vi "Initialize Addon.vi"(8 "error in (no error)":errorcluster, 11 "Cluster":T19={"J1939 XNET Settings"={"XNET Database"="", "XNET Cluster"="", "CAN Port"="", "Baud rate [Bd]"=0, "Termination"=0, "Incoming Rate"=0, "Outcoming Rate"=0, "Write Decimation"=1}, "Incoming Decimation"=0, "Outgoing Decimation"=0, {"RT Bitfile Path"=path "", "RIO Device"=0, "Enable"=FALSE}, "Incoming Single Point Configuraiton"={"Incoming Single Point Frame"={"ID"=[], "Channel Array Positions"=[], "Frame Length"=[], "Frame Channels"=[]}, "Channel Pairs"={"Chan Refs"=[], "Previous Chan Values"=[]}, "# of Channels"=0, "Name"=""}, "Outgoing Cyclic Configuraiton"={"Outgoing Cyclic Frame"={"ID"=[], "Channel Array Positions"=[], "Frame Length"=[], "Transmit Propreties"=[], "Frame Channels"=[]}, "Channel Pairs"={"Block Data Refs"=[], "Previous Chan Values"=[]}, "Name"=""}, "Internal Command Engine References"={"Response Refs"={"Block Data Refs"=[], "Values Array"=[], "# of Channels"=0, "Name"=""}, "Command Refs"={"Block Data Refs"=[], "Values Array"=[], "# of Channels"=0, "Name"=""}, "Command Names"=[], "Response Names"=[]}, "FPGA Bitfile Settings"={"RT Bitfile Path"=path "", "RIO Device"=0, "Enable"=FALSE}, "J1939 Monitor Settings"={"J1939 Network Address"=0, "Name"=0}, "Simulated Addresses"=[]} {"Simulated Addresses"."J1939 XNET Settings"."Name" format="%.0x"; "Simulated Addresses"."DM1 Data"."Data Reference" format="%.0x"; "Simulated Addresses"."DM1 Active?"."Data Reference" format="%.0x"; "Simulated Addresses"."DM2 Data"."Data Reference" format="%.0x"; "Simulated Addresses"."DM2 Active?"."Data Reference" format="%.0x"; "J1939 Monitor Settings"."Name" format="%.0x"; "J1939 XNET Settings"."Termination" items=["Off", "On"]; "Incoming Single Point Configuraiton"."Channel Pairs"."Chan Refs" format="%.0x"; "Outgoing Cyclic Configuraiton"."Outgoing Cyclic Frame"."Transmit Propreties"."Transmit Time" format="%#_p"; "Outgoing Cyclic Configuraiton"."Channel Pairs"."Block Data Refs"."Data Reference" format="%.0x"; "Internal Command Engine References"."Response Refs"."Block Data Refs" format="%.0x"; "Internal Command Engine References"."Command Refs"."Block Data Refs"."Data Reference" format="%.0x"}) -> (0 "error out":errorcluster, 3 "cluster":T1={"Device Error"={"status"=FALSE, "code"=0, "source"=""}, "VI Refs"=[], "Error Handling Cluster"={"Error Process Q"=refnum, "Process Qs"=[]}, "J1939 Process Parameters"={"J1939 XNET Settings"={"XNET Database"="", "XNET Cluster"="", "CAN Port"="", "Baud rate [Bd]"=0, "Termination"=0, "Incoming Rate"=0, "Outcoming Rate"=1, "Write Decimation"=1}, "Incoming Single Point Configuraiton"={"Incoming Single Point Frame"={"ID"=[], "Conversion"=[], "Channel Array Positions"=[], "Frame Length"=[]}, "Channel Pairs"={"Chan Refs"=[], "Previous Chan Values"=[]}, "Read FIFO"=refnum}, "Outgoing Cyclic Configuraiton"={"Outgoing Cyclic Frame"={"ID"=[], "Conversion"=[], "Channel Array Positions"=[], "Frame Length"=[], "Transmit Propreties"=[]}, "Channel Pairs"={"Block Data Refs"=[], "Previous Chan Values"=[]}, "Write FIFO"=refnum}, "J1939 Monitor Settings"={"J1939 Network Address"=0, "Name"=0}, "Simulated Addresses"=[], "Simulated Addresses LUT"=variant}, "Internal Command Engine References"={"Response Refs"={"Block Data Refs"=[], "Values Array"=[]}, "Command Refs"={"Block Data Refs"=[], "Values Array"=[]}, "Response HW_Internal Cmds"=refnum, "Command HW_Internal Cmds"=refnum, "Command Names"=[], "Response Names"=[]}, "FPGA Session"=0, "Incoming Decimation"=0, "Outgoing Decimation"=0} {"Internal Command Engine References"."Command Refs"."Block Data Refs"."Data Reference" format="%.0x"; "Internal Command Engine References"."Response Refs"."Block Data Refs" format="%.0x"; "J1939 Process Parameters"."Simulated Addresses"."Simulated Addresses"."J1939 XNET Settings"."Name" format="%.0x"; "J1939 Process Parameters"."J1939 Monitor Settings"."Name" format="%.0x"; "J1939 Process Parameters"."Outgoing Cyclic Configuraiton"."Channel Pairs"."Block Data Refs"."Data Reference" format="%.0x"; "J1939 Process Parameters"."Outgoing Cyclic Configuraiton"."Outgoing Cyclic Frame"."Transmit Propreties"."Transmit Time" format="%#_p"; "J1939 Process Parameters"."J1939 XNET Settings"."Termination" items=["Off", "On"]; "J1939 Process Parameters"."Incoming Single Point Configuraiton"."Channel Pairs"."Chan Refs" format="%.0x"})   [LabVIEW 2013, in "J1939 Addon Engine.lvlib"]
uses:
  J1939 Addon Engine.lvlib
  Shared/Types/Compile Addon Settings.ctl
  Shared/Types/XNET Settings.ctl
  Shared/Types/SysDef FPGA Settings.ctl
  Shared/Types/SysDef Incoming Single Point Configurations.ctl
  Shared/Types/SysDef Incoming Frame Configuration.ctl
  Types/Incoming Single Point Channel Pairs.ctl
  <vilib>/NI Veristand/Custom Device API/Data Reference.ctl
  Shared/Types/SysDef Outgoing Cyclic Configurations.ctl
  Shared/Types/SysDef Outgoing Frame Configuration.ctl
  Shared/Types/XNET Frame Event Properties.ctl
  Types/Outgoing Cyclic Channel Pairs.ctl
  <vilib>/NI Veristand/Custom Device API/Block Data Reference.ctl
  Shared/Types/SysDef Command Settings.ctl
  Shared/Types/Monitor Settings.ctl
  Shared/Types/Compiled Simulated Settings.ctl
  Types/Inline Device Cluster.ctl
  Error Handling API/Controls/Error Handling Cluster.ctl
  Types/Process Parameters.ctl
  Types/Incoming Single Point Configuration.ctl
  Types/Incoming Single Point Frame Pairs.ctl
  Types/Outgoing Cyclic Configuration.ctl
  Types/Outgoing Cyclic Frame Pairs.ctl
  Types/Simulated Settings.ctl
  Types/DTC FIFOs.ctl
  Types/Internal Command Configuration Parameters.ctl
  <vilib>/NI Veristand/Custom Device API/Custom Device API.lvlib
  Shared/J1939 Addon Shared.lvlib
  Error Handling API/Error Handling API.lvlib
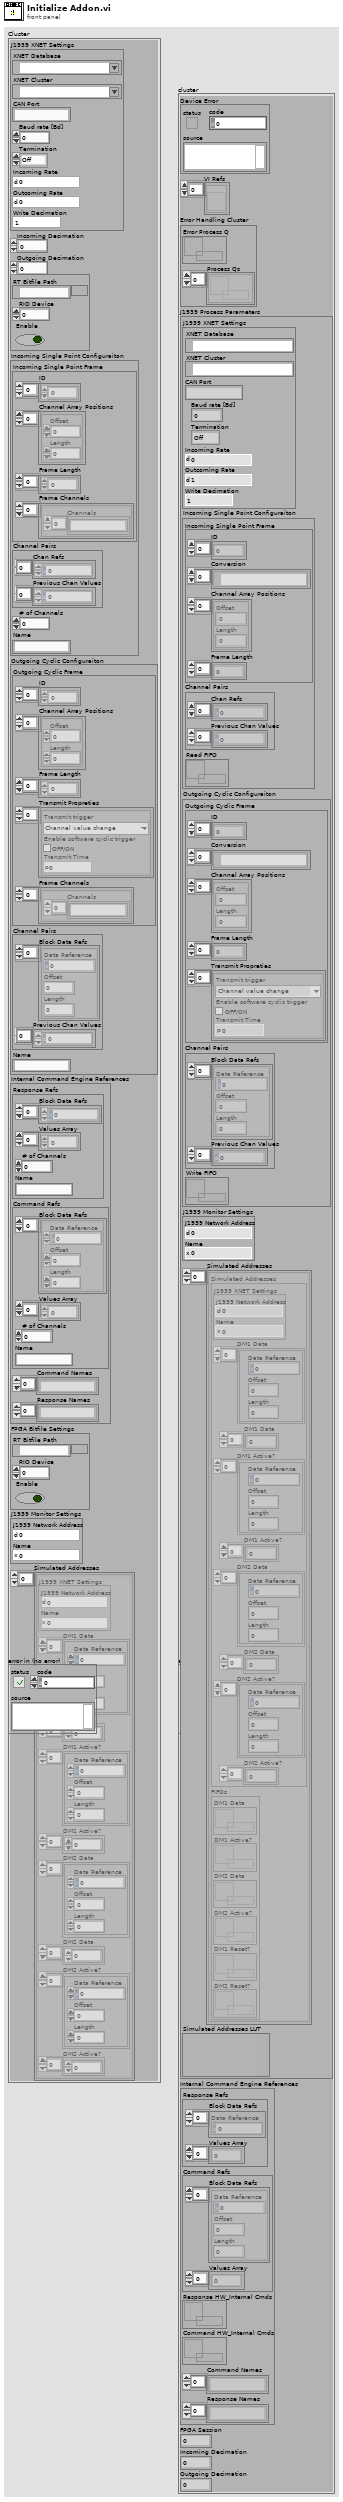
[diagram p1: front panel]
types:
  T1 = typedef "J1939 Addon Engine.lvlib/Inline Device Cluster.ctl" = cluster{"Device Error":errorcluster, "VI Refs":refnum<vi>[], "Error Handling Cluster":T2, "J1939 Process Parameters":T3, "Internal Command Engine References":T18, "FPGA Session":u32, "Incoming Decimation":u32, "Outgoing Decimation":u32}
  T2 = typedef "J1939 Addon Engine.lvlib/Error Handling API.lvlib/Error Handling Cluster.ctl" = cluster{"Error Process Q":refnum<queue>, "Process Qs":refnum<queue>[]}
  T3 = typedef "J1939 Addon Engine.lvlib/Process Parameters.ctl" = cluster{"J1939 XNET Settings":T4, "Incoming Single Point Configuraiton":T5, "Outgoing Cyclic Configuraiton":T9, "J1939 Monitor Settings":T14, "Simulated Addresses":T15[], "Simulated Addresses LUT":variant}
  T4 = typedef "J1939 Addon Shared.lvlib/XNET Settings.ctl" = cluster{"XNET Database":refnum<k21>, "XNET Cluster":refnum<k21>, "CAN Port":string, "Baud rate [Bd]":u32, "Termination":u32, "Incoming Rate":u32, "Outcoming Rate":u32, "Write Decimation":u32}
  T5 = typedef "J1939 Addon Engine.lvlib/Incoming Single Point Configuration.ctl" = cluster{"Incoming Single Point Frame":T6, "Channel Pairs":T7, "Read FIFO":refnum<k33>}
  T6 = typedef "J1939 Addon Engine.lvlib/Incoming Single Point Frame Pairs.ctl" = cluster{"ID":u32[], "Conversion":refnum<k21>[], "Channel Array Positions":cluster{"Offset":u32, "Length":u32}[], "Frame Length":u32[]}
  T7 = typedef "J1939 Addon Engine.lvlib/Incoming Single Point Channel Pairs.ctl" = cluster{"Chan Refs":T8[], "Previous Chan Values":dbl[]}
  T8 = typedef "Custom Device API.lvlib/Data Reference.ctl" = i32
  T9 = typedef "J1939 Addon Engine.lvlib/Outgoing Cyclic Configuration.ctl" = cluster{"Outgoing Cyclic Frame":T10, "Channel Pairs":T12, "Write FIFO":refnum<k33>}
  T10 = typedef "J1939 Addon Engine.lvlib/Outgoing Cyclic Frame Pairs.ctl" = cluster{"ID":u32[], "Conversion":refnum<k21>[], "Channel Array Positions":cluster{"Offset":u32, "Length":u32}[], "Frame Length":u32[], "Transmit Propreties":T11[]}
  T11 = typedef "J1939 Addon Shared.lvlib/XNET Frame Event Properties.ctl" = cluster{"Transmit trigger":enum16{"Channel value change"}, "Enable software cyclic trigger":bool, "Transmit Time":dbl}
  T12 = typedef "J1939 Addon Engine.lvlib/Outgoing Cyclic Channel Pairs.ctl" = cluster{"Block Data Refs":T13[], "Previous Chan Values":dbl[]}
  T13 = typedef "Custom Device API.lvlib/Block Data Reference.ctl" = cluster{"Data Reference":T8, "Offset":i32, "Length":i32}
  T14 = typedef "J1939 Addon Shared.lvlib/Monitor Settings.ctl" = cluster{"J1939 Network Address":u8, "Name":u64}
  T15 = typedef "J1939 Addon Engine.lvlib/Simulated Settings.ctl" = cluster{"Simulated Addresses":T16, "FIFOs":T17}
  T16 = typedef "J1939 Addon Shared.lvlib/Compiled Simulated Settings.ctl" = cluster{"J1939 XNET Settings":T14, "DM1 Data":T13[], "DM1 Data":dbl[], "DM1 Active?":T13[], "DM1 Active?":dbl[], "DM2 Data":T13[], "DM2 Data":dbl[], "DM2 Active?":T13[], "DM2 Active?":dbl[]}
  T17 = typedef "J1939 Addon Engine.lvlib/DTC FIFOs.ctl" = cluster{"DM1 Data":refnum<k33>, "DM1 Active?":refnum<k33>, "DM2 Data":refnum<k33>, "DM2 Active?":refnum<k33>, "DM1 Reset?":refnum<k33>, "DM2 Reset?":refnum<k33>}
  T18 = typedef "J1939 Addon Engine.lvlib/Internal Command Configuration Parameters.ctl" = cluster{"Response Refs":cluster{"Block Data Refs":T8[], "Values Array":dbl[]}, "Command Refs":cluster{"Block Data Refs":T13[], "Values Array":dbl[]}, "Response HW_Internal Cmds":refnum<k33>, "Command HW_Internal Cmds":refnum<k33>, "Command Names":string[], "Response Names":string[]}
  T19 = typedef "J1939 Addon Shared.lvlib/Compile Addon Settings.ctl" = cluster{"J1939 XNET Settings":T4, "Incoming Decimation":u32, "Outgoing Decimation":u32, T20, "Incoming Single Point Configuraiton":T21, "Outgoing Cyclic Configuraiton":T23, "Internal Command Engine References":T25, "FPGA Bitfile Settings":T20, "J1939 Monitor Settings":T14, "Simulated Addresses":T16[]}
  T20 = typedef "J1939 Addon Shared.lvlib/SysDef FPGA Settings.ctl" = cluster{"RT Bitfile Path":path, "RIO Device":u16, "Enable":bool}
  T21 = typedef "J1939 Addon Shared.lvlib/SysDef Incoming Single Point Configurations.ctl" = cluster{"Incoming Single Point Frame":T22, "Channel Pairs":T7, "# of Channels":u32, "Name":string}
  T22 = typedef "J1939 Addon Shared.lvlib/SysDef Incoming Frame Configuration.ctl" = cluster{"ID":u32[], "Channel Array Positions":cluster{"Offset":u32, "Length":u32}[], "Frame Length":u32[], "Frame Channels":cluster{"Channels":string[]}[]}
  T23 = typedef "J1939 Addon Shared.lvlib/SysDef Outgoing Cyclic Configurations.ctl" = cluster{"Outgoing Cyclic Frame":T24, "Channel Pairs":T12, "Name":string}
  T24 = typedef "J1939 Addon Shared.lvlib/SysDef Outgoing Frame Configuration.ctl" = cluster{"ID":u32[], "Channel Array Positions":cluster{"Offset":u32, "Length":u32}[], "Frame Length":u32[], "Transmit Propreties":T11[], "Frame Channels":cluster{"Channels":string[]}[]}
  T25 = typedef "J1939 Addon Shared.lvlib/SysDef Command Settings.ctl" = cluster{"Response Refs":cluster{"Block Data Refs":T8[], "Values Array":dbl[], "# of Channels":u32, "Name":string}, "Command Refs":cluster{"Block Data Refs":T13[], "Values Array":dbl[], "# of Channels":u32, "Name":string}, "Command Names":string[], "Response Names":string[]}
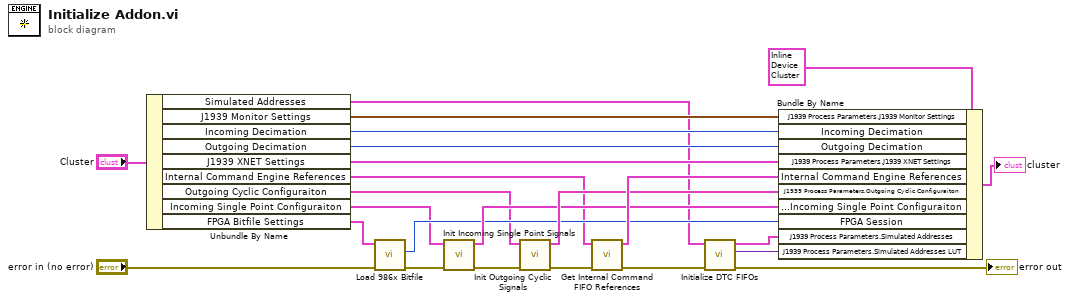
[diagram p0: block diagram]
diagram:
  n1 = Unbundle By Name("Cluster") -> ("Simulated Addresses"=w3:T16[], "J1939 Monitor Settings"=w6:T14, "Incoming Decimation"=w19:u32, "Outgoing Decimation"=w20:u32, "J1939 XNET Settings"=w13:T4, "Internal Command Engine References"=w18:T25, "Outgoing Cyclic Configuraiton"=w17:T23, "Incoming Single Point Configuraiton"=w16:T21, "FPGA Bitfile Settings"=w14:T20)
  n2 = call "Load 986x Bitfile.vi"("error in (no error)"="error in (no error)", "FPGA Settings"=w14) -> ("error out"=w15:errorcluster, "FPGA Session"=w21:u32)  [unwired: 8 in]
  n3 = call "Init Incoming Single Point Signals.vi"("error in"=w15, "Incoming Single Point Configuraiton"=w16) -> ("error out"=w8:errorcluster, "Incoming Single Point Configuraiton"=w22:T5)  [unwired: 8 in]
  n4 = call "Init Outgoing Cyclic Signals.vi"("error in"=w8, "Outgoing Cyclic Configuraiton"=w17) -> ("error out"=w10:errorcluster, "Outgoing Cyclic Configuraiton"=w23:T9)  [unwired: 8 in]
  n5 = call "Get Internal Command FIFO References.vi"("error in (no error)"=w10, "Internal Command Engine References"=w18) -> ("error out"=w5:errorcluster, "Internal Command Engine References"=w24:T18)  [unwired: 8 in]
  n6 = call "Initialize DTC FIFOs.vi"("error in"=w5, "Simulated Addresses"=w3) -> ("error out"=→"error out":errorcluster, "Simulated Addresses LUT"=w2:variant, "Simulated Addresses"=w1:T15[])  [unwired: 7 in]
  n7 = Bundle By Name(cluster=T1 {"Device Error"={"status"=FALSE, "code"=0, "source"=""}, "VI Refs"=[], "Error Handling Cluster"={"Error Process Q"=refnum, "Process Qs"=[]}, "J1939 Process Parameters"={"J1939 XNET Settings"={"XNET Database"="", "XNET Cluster"="", "CAN Port"="", "Baud rate [Bd]"=0, "Termination"=0, "Incoming Rate"=0, "Outcoming Rate"=0, "Write Decimation"=0}, "Incoming Single Point Configuraiton"={"Incoming Single Point Frame"={"ID"=[], "Conversion"=[], "Channel Array Positions"=[], "Frame Length"=[]}, "Channel Pairs"={"Chan Refs"=[], "Previous Chan Values"=[]}, "Read FIFO"=refnum}, "Outgoing Cyclic Configuraiton"={"Outgoing Cyclic Frame"={"ID"=[], "Conversion"=[], "Channel Array Positions"=[], "Frame Length"=[], "Transmit Propreties"=[]}, "Channel Pairs"={"Block Data Refs"=[], "Previous Chan Values"=[]}, "Write FIFO"=refnum}, "J1939 Monitor Settings"={"J1939 Network Address"=0, "Name"=0}, "Simulated Addresses"=[], "Simulated Addresses LUT"=variant}, "Internal Command Engine References"={"Response Refs"={"Block Data Refs"=[], "Values Array"=[]}, "Command Refs"={"Block Data Refs"=[], "Values Array"=[]}, "Response HW_Internal Cmds"=refnum, "Command HW_Internal Cmds"=refnum, "Command Names"=[], "Response Names"=[]}, "FPGA Session"=0, "Incoming Decimation"=0, "Outgoing Decimation"=0}, "J1939 Process Parameters.J1939 Monitor Settings"=w6, "Incoming Decimation"=w19, "Outgoing Decimation"=w20, "J1939 Process Parameters.J1939 XNET Settings"=w13, "Internal Command Engine References"=w24, "J1939 Process Parameters.Outgoing Cyclic Configuraiton"=w23, "J1939 Process Parameters.Incoming Single Point Configuraiton"=w22, "FPGA Session"=w21, "J1939 Process Parameters.Simulated Addresses"=w1, "J1939 Process Parameters.Simulated Addresses LUT"=w2) -> (→"cluster":T1)
